vi "Write_csv_with_Headders.vi"(11 "file path (dialog if empty)":path) -> (0 "error out":errorcluster, 3 "File Path":path)   [LabVIEW 2024]
uses:
  <vilib>/Utility/file.llb/Write Delimited Spreadsheet (string).vi
panel:
  out "string":string
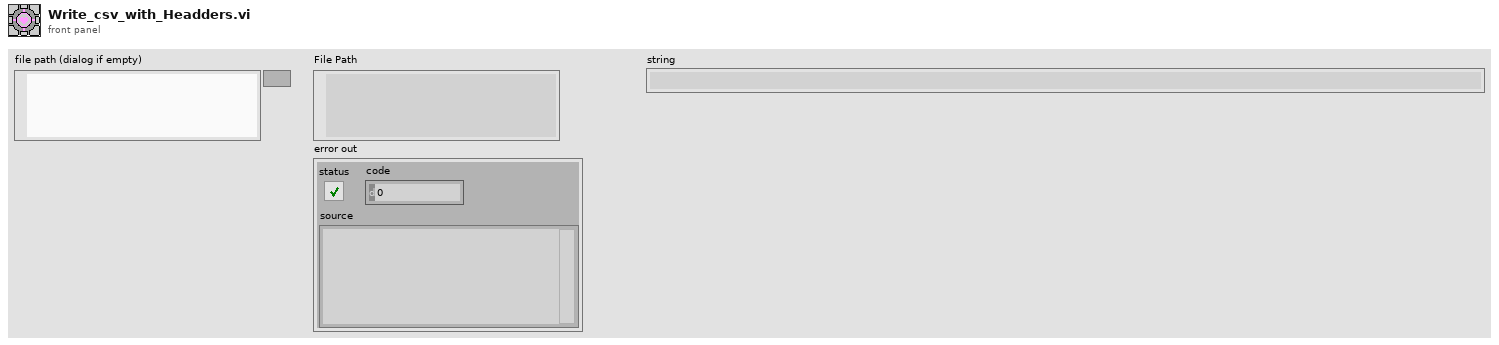
[diagram p1: front panel]
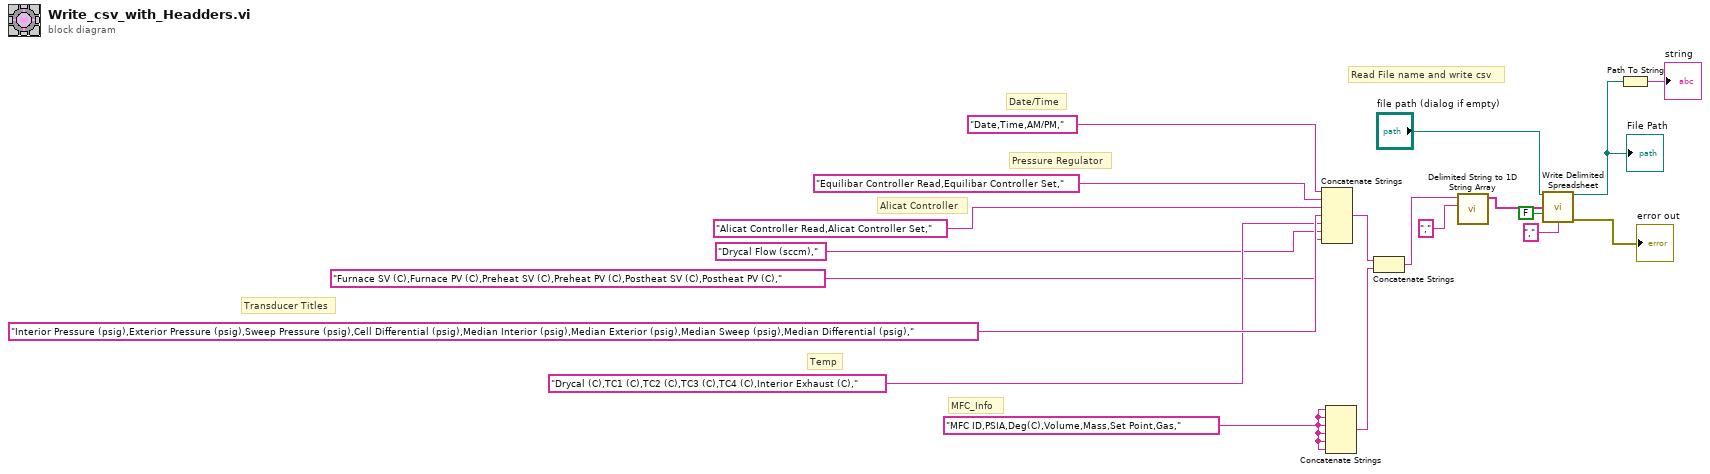
[diagram p0: block diagram]
diagram:
  w3 = "MFC ID,PSIA,Deg(C),Volume,Mass,Set Point,Gas,"
  # "Alicat Controller"
  # "Temp"
  # "Date/Time"
  # "Transducer Titles"
  # "Pressure Regulator"
  # "Read File name and write csv"
  # "MFC_Info"
  n1 = Concatenate Strings("Date,Time,AM/PM," ("string"), "Equilibar Controller Read,Equilibar Controller Set," ("string"), "Alicat Controller Read,Alicat Controller Set," ("string"), "Interior Pressure (psig),Exterior Pressure (psig),Sweep Pressure (psig),Cell Differential (psig),Median Interior (psig),Median Exterior (psig),Median Sweep (psig),Median Differential (psig)," ("string"), "Drycal (C),TC1 (C),TC2 (C),TC3 (C),TC4 (C),Interior Exhaust (C)," ("string"), "Drycal Flow (sccm)," ("string"), "Furnace SV (C),Furnace PV (C),Preheat SV (C),Preheat PV (C),Postheat SV (C),Postheat PV (C)," ("string")) -> (w8:string)
  n2 = Concatenate Strings(w3, w3, w3, w3, w3, w3) -> (w10:string)
  n3 = Concatenate Strings(w8, w10) -> (w9:string)
  n4 = call <vilib>:"Delimited String to 1D String Array.vi"("delimiter"=",", "delimited string"=w9) -> ("string array"=w18:string[])  [unwired: 9 in]
  n5 = call-poly <vilib>:"Write Delimited Spreadsheet.vi"("file path (dialog if empty)"="file path (dialog if empty)", "1D data"=w18, "append to file? (new file:F)"=FALSE, "delimiter (\\t)"="," ("delimiter (\\t)")) -> ("new file path (Not A Path if cancelled)"=w14:path, "error out"=→"error out":errorcluster)  [unwired: 10 in]
  "File Path" <- w14
  n6 = Path To String(path=w14) -> (string=→"string":string)
